vi "Meas_freq.vi"(1 "source":tag, 2 "edge":i32(ring)=10280 items=["Rising"=10280, "Falling"=10171], 3 "Time miliseconds":u32, 4 "counter":tag) -> (0 "?":dbl(graph))   [LabVIEW 2024]
uses:
  <vilib>/Utility/error.llb/DialogType.ctl
  <vilib>/DAQmx/read.llb/DAQmx Read (Counter DBL 1Chan 1Samp).vi
  <vilib>/DAQmx/create/channels.llb/DAQmx Create Channel (CI-Count Edges).vi
  <vilib>/DAQmx/miscellaneous.llb/DAQmx Fill In Error Info.vi
  <resource>/objmgr/daqmx.rc
panel:
  in  "Stop":bool
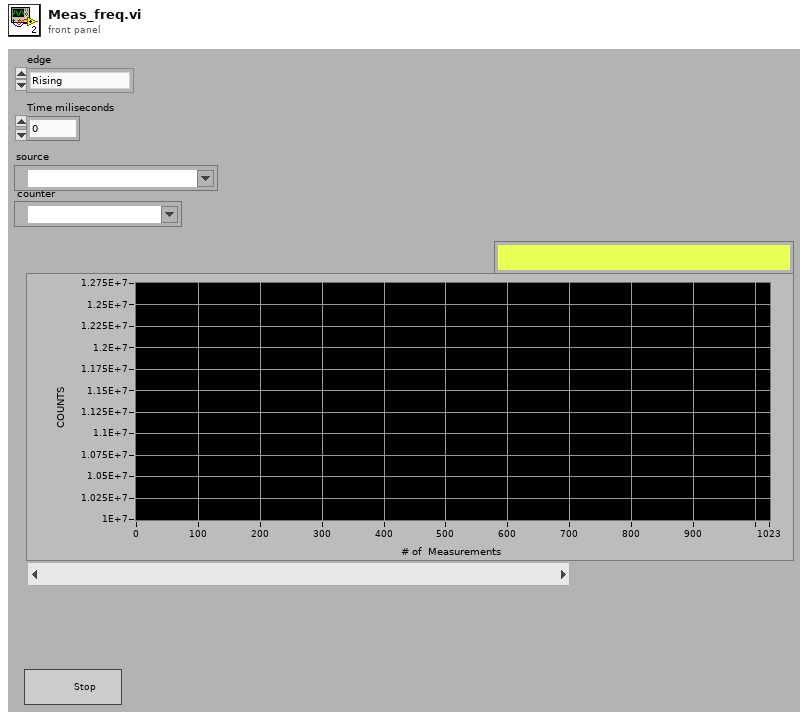
[diagram p1: front panel]
types:
  T1 = typedef "DialogType.ctl" = u16
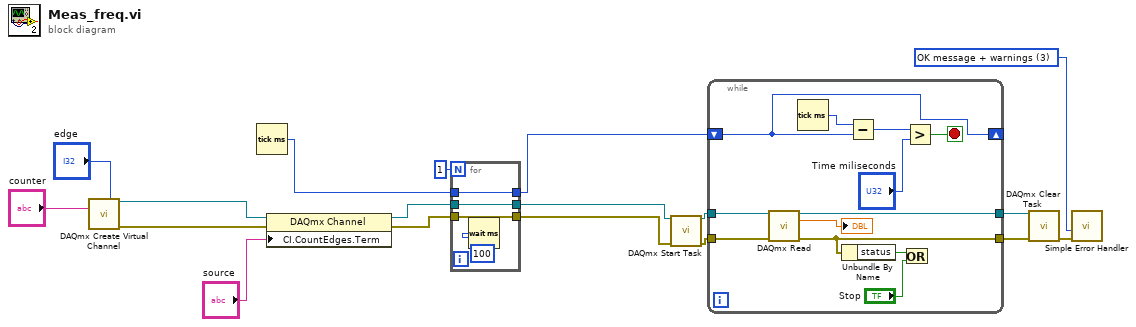
[diagram p0: block diagram]
diagram:
  w13 = T1 3 items=["no dialog", "OK message", "continue or stop message", "OK message + warnings", "continue/stop + warnings"] ("type of dialog (OK msg:1)")
  n1 = call-poly <vilib>:"DAQmx Create Virtual Channel.vi"("edge"="edge", "counter"="counter") -> ("task out"=w17:refnum<k21>, "error out"=w16:errorcluster)  [unwired: 12 in]
  n2 = Tick Count (ms)() -> (millisecond timer value=w7:u32)
  n3 = property class="DAQmx Channel"(reference=w17, error in=w16, "CI.CountEdges.Term"="source") -> (reference out=w4:refnum<k21>, error out=w2:errorcluster)
  n4 = for {
    N: 1 -> [_]
    tunnel: w7 -> [w20]
    tunnel: [w20] -> w6
    tunnel: [w22] -> w5
    tunnel: w4 -> [w22]
    tunnel: w2 -> [w21]
    tunnel: [w21] -> w3
    n5 = Wait (ms)(milliseconds to wait=u32 100 ("millisecond timer value")) -> ()  [unwired: 1 out]
  }
  n6 = call <vilib>:"DAQmx Start Task.vi"("task/channels in"=w5, "error in"=w3) -> ("task out"=w11:refnum<k21>, "error out"=w9:errorcluster)  [unwired: 12 in]
  n7 = while {
    tunnel: [w31] -> w12
    tunnel: w11 -> [w30]
    tunnel: w9 -> [w29]
    tunnel: [w28] -> w10
    shift-right: [w23] -> _
    shift-left: w6 -> [w23]
    stop <- w25 stop-if-true
    n8 = call-poly <vilib>:"DAQmx Read.vi"("task/channels in"=w30, "error in"=w29) -> ("task out"=w31:refnum<k21>, "data"=→"?":dbl, "error out"=w28:errorcluster)  [unwired: 11 in]
    n9 = Tick Count (ms)() -> (millisecond timer value=w27:u32)
    n10 = Unbundle By Name(w28) -> ("status"=w33:bool)
    n11 = Subtract(x=w27, y=w23) -> (x-y=w24:u32)
    n12 = Or(x=w33, y="Stop") -> ()  [unwired: 1 out]
    n13 = Greater?(x=w24, y="Time miliseconds") -> (0:w25:bool)
  }
  n14 = call <vilib>:"DAQmx Clear Task.vi"("task in"=w12, "error in"=w10) -> ("error out"=w14:errorcluster)  [unwired: 13 in]
  n15 = call <vilib>:"Simple Error Handler.vi"("type of dialog (OK msg:1)"=w13, "error in (no error)"=w14) -> ()  [unwired: 3 in, 5 out]
